vi "PH_PILS.vis LaserPowerOnKnob.vi"(0 "i ref in":refnum<vi>, 5 "error IO":errorcluster) -> (14 "i ref out":refnum<vi>, 19 "error out":errorcluster)   [LabVIEW 2014, in "PH_PILS.lvlib"]
uses:
  PH_PILS.lvlib
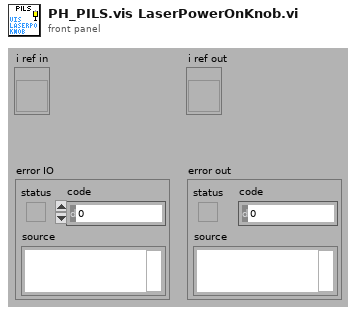
[diagram p1: front panel]
types:
  T1 = typedef "PH_PILS.lvlib/PH_PILS.i attribute.ctl" = cluster{"Boolean":cluster{"GUI Ref":refnum<vi>, "Status":i32}[], "GUI Refs Exp. Shutters":cluster{"1":refnum<vi>, "2":refnum<vi>, "3":refnum<vi>, "4":refnum<vi>}, "Tristate2Run GUI Refs":refnum<vi>[], "EO-Likes":cluster{"GUI Ref":refnum<vi>, "Status":i32}[], "Operation Mode":cluster{"Operation Mode":T2, "GUI":cluster{"Ref State":refnum<vi>, "Ref":refnum<vi>}, "Servicemode":cluster{"Tagname":string, "Status":i32}, "Labormode":cluster{"Tagname":string, "Status":i32}, "Searchmode":cluster{"Tagname":string, "Status":i32}, "Shotmode":cluster{"Tagname":string, "Status":i32}}, "Submode":cluster{"Submode":T3, "GUI":cluster{"Ref State":refnum<vi>, "Ref":refnum<vi>}, "Submode":cluster{"Tagname":string, "Status":i32}}, "Experiment":cluster{"Experiment":enum16{"unknown", "intern", "4 (Z6)", "3", "2", "1"}, "GUI":cluster{"Ref State":refnum<vi>, "Ref":refnum<vi>}, "intern":cluster{"Tagname":string, "Status":i32}, "Exp 4":cluster{"Tagname":string, "Status":i32}, "Exp 3":cluster{"Tagname":string, "Status":i32}, "Exp 2":cluster{"Tagname":string, "Status":i32}, "Exp 1":cluster{"Tagname":string, "Status":i32}}, "TristateNormal":cluster{"GUI Ref":refnum<vi>, "Status":i32}[], "Door Tags":cluster{"GUI Ref":refnum<vi>, "Status":i32}[], "GUIlessTags":cluster{"Name":string, "Status":i32}[], "Beamline GUI Refs":refnum<vi>[], "Special Boolean":cluster{"GUI Ref":refnum<vi>, "Status":i32}[], "Laserpower":cluster{"GUI Ref":refnum<vi>, "Status":i32}[], "Shutter":cluster{"GUI Ref":refnum<vi>, "Status":i32}[], "Tristate EO Like":cluster{"GUI Ref":refnum<vi>, "Status":i32}[], "PP":cluster{"GUI Ref":refnum<vi>, "Status":i32, "Head Ref":refnum<vi>, "Slider Ref":refnum<vi>}[], "Switch Knobs":cluster{"GUI Ref":refnum<vi>, "Status":i32}[], "Latch Knob GUI Refs":refnum<vi>[], "FailureCounter":i32, "Enabled Status":cluster{"Laser":i32, "PreAmp":i32, "MainAmp":i32}, "Mercury":refnum<vi>, "Instance Rods":string, "Logfile":path, "Beckhoff-Instance Internal":string, "Beckhoff-Instance External":string, "Enabling Rights":cluster{"Name":string, "Password":string, "PA?":bool, "MA?":bool, "Exp?":bool}[]}
  T2 = typedef "PH_PILS.lvlib/PH_PILS.Operation Mode.ctl" = enum16{"unknown", "Service", "Labor", "Search", "Shot"}
  T3 = typedef "PH_PILS.lvlib/PH_PILS.Submode.ctl" = enum16{"unknown", "HV-Normal", "HV-Test"}
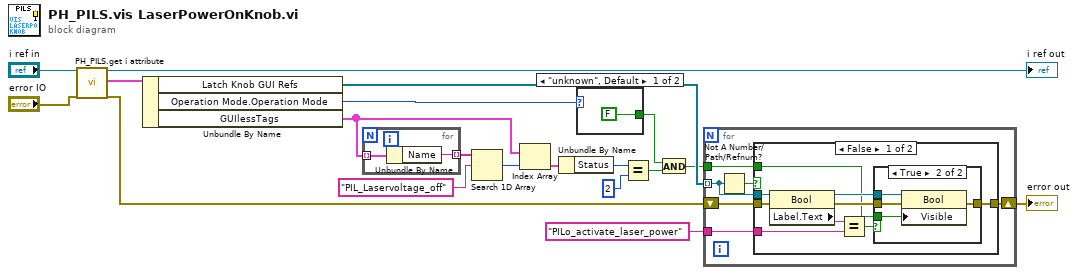
[diagram p0: block diagram]
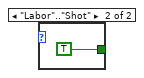
[diagram p2: hidden frame]
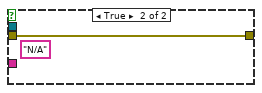
[diagram p4: hidden frame]
diagram:
  n1 = call "PH_PILS.get i attribute.vi"("i ref in"="i ref in", "error in (no error)"="error IO") -> ("i ref out"=→"i ref out":refnum<vi>, "i attribute"=w16:T1, "error out"=w14:errorcluster)  [unwired: 15 in]
  n2 = Unbundle By Name(w16) -> ("Latch Knob GUI Refs"=w15:refnum<vi>[], "Operation Mode.Operation Mode"=w5:T2, "GUIlessTags"=w4:cluster{"Name":string, "Status":i32}[])
  n3 = for {
    tunnel: w4 -> [w21] mode=indexing
    tunnel: [w20] -> w11 mode=indexing
    n4 = Unbundle By Name(w21) -> ("Name"=w20:string)
  }
  n5 = Search 1D Array(1D array=w11, element="PIL_Laservoltage_off") -> (index of element=w9:i32)  [unwired: 1 in]
  n6 = Index Array(array=w4, index=w9) -> (element=w8:cluster{"Name":string, "Status":i32})
  n7 = Unbundle By Name(w8) -> ("Status"=w7:i32)
  n8 = case shown="\"unknown\", Default" w5 {
    tunnel: [FALSE TRUE] -> w3
    frame "unknown", Default {
    }
    frame "Labor".."Shot" {
    }
  }
  n9 = Equal?(x=w7, y=2) -> (x = y?=w2:bool)
  n10 = And(x=w3, y=w2) -> (x .and. y?=w1:bool)
  n11 = for {
    tunnel: w15 -> [w26] mode=indexing
    shift-right: [w27] -> w12
    shift-left: w14 -> [w29]
    tunnel: "PILo_activate_laser_power" -> [w25]
    tunnel: w1 -> [w24]
    n12 = Not A Number/Path/Refnum?(number/path/refnum=w26) -> (NaN/Path/Refnum?=w28:bool)
    n13 = case shown="False" w28 {
      tunnel: w26 -> [w38 _]
      tunnel: w29 -> [w37 w44]
      tunnel: [w33 w44] -> w27
      tunnel: w25 -> [w35 _]
      tunnel: w24 -> [w30 _]
      frame False {
        n14 = property class="Bool"(reference=w38, error in=w37) -> (reference out=w32:refnum<vi>, error out=w34:errorcluster, "Label.Text"=w36:string)
        n15 = Equal?(x=w36, y=w35) -> (x = y?=w31:bool)
        n16 = case shown="True" w31 {
          tunnel: w34 -> [w39 w43]
          tunnel: [w39 w42] -> w33
          tunnel: w32 -> [_ w41]
          tunnel: w30 -> [_ w40]
          frame False {
          }
          frame True {
            n17 = property class="Bool"(reference=w41, error in=w43, "Visible"=w40) -> (error out=w42:errorcluster)  [unwired: 1 out]
          }
        }
      }
      frame True {
        (unwired) "N/A" ("Label.Text")
      }
    }
  }
  "error out" <- w12
